vi "Untitled 3.vi"() -> ()   [LabVIEW 2016]
panel:
  in  "stop":bool
  out "result":bool
  in  "new element/subarray":bool
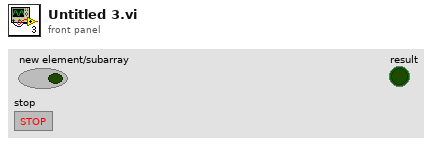
[diagram p1: front panel]
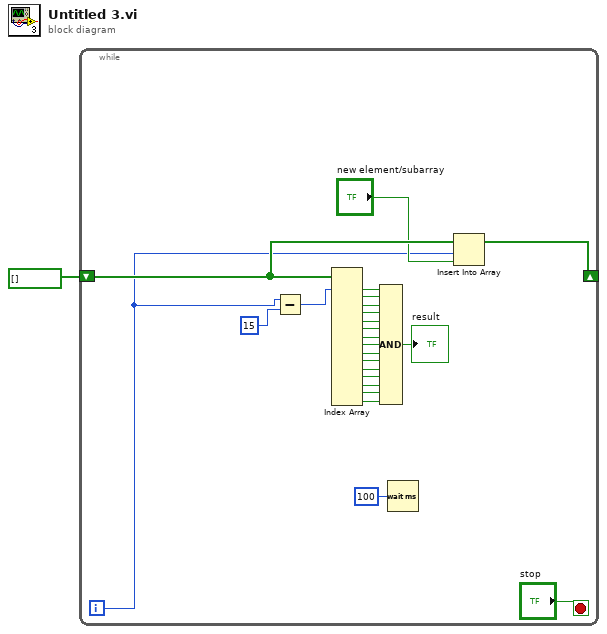
[diagram p0: block diagram]
diagram:
  n1 = while {
    shift-right: [w10] -> _
    shift-left: bool[] [] ("array") -> [w9]
    i -> [w4]
    stop <- "stop" stop-if-true
    n2 = Subtract(x=w4, y=15) -> (x-y=w5:i32)
    n3 = Index Array(array=w9, index #1=w5) -> (element #1=w25:bool, element #2=w24:bool, element #3=w23:bool, element #4=w22:bool, element #5=w21:bool, element #6=w20:bool, element #7=w19:bool, element #8=w18:bool, element #9=w17:bool, element #10=w16:bool, element #11=w15:bool, element #12=w14:bool, element #13=w13:bool, element #14=w12:bool, element #15=w11:bool)  [unwired: 14 in]
    n4 = Compound Arithmetic op=AND(w25, w24, w23, w22, w21, w20, w19, w18, w17, w16, w15, w14, w13, w12, w11) -> (→"result":bool)
    n5 = Wait (ms)(milliseconds to wait=u32 100) -> ()  [unwired: 1 out]
    n6 = Insert Into Array(array=w9, index=w4, new element="new element/subarray") -> (w10:bool[])
  }
